vi "InicializaciónMF.vi"(1 "Lista de Direcciones":i16[](array[numeric])) -> (0 "error out 2":errorcluster)   [LabVIEW 2015]
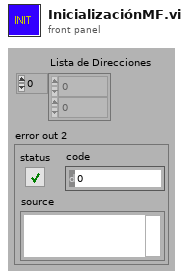
[diagram p1: front panel]
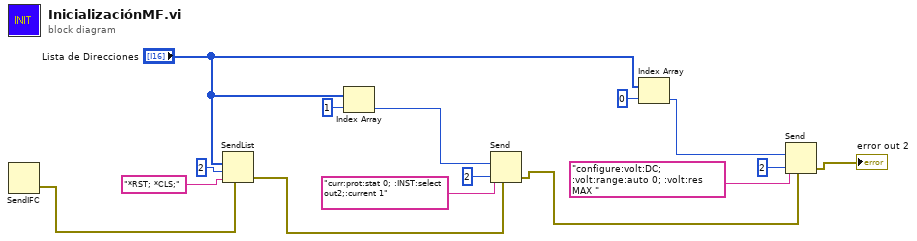
[diagram p0: block diagram]
diagram:
  n1 = SendIFC() -> (0:w10:errorcluster)  [unwired: 2 in, 1 out]
  n2 = SendList(2:"Lista de Direcciones", 3:u8 2, 4:w10, 5:"*RST; *CLS;") -> (8:w8:errorcluster)  [unwired: 1 in, 2 out]
  n3 = Index Array(array="Lista de Direcciones", index=1) -> (element=w11:i16)
  n4 = Send(2:w11, 3:i16 2 ("mode"), 4:w8, 5:"curr:prot:stat 0; :INST:select out2;:current 1") -> (8:w4:errorcluster)  [unwired: 1 in, 2 out]
  n5 = Index Array(array="Lista de Direcciones", index=0) -> (element=w2:i16)
  n6 = Send(2:w2, 3:i16 2 ("mode"), 4:w4, 5:"configure:volt:DC; :volt:range:auto 0; :volt:res MAX ") -> (8:→"error out 2":errorcluster)  [unwired: 1 in, 2 out]
